vi "WorkorderHandler_LockedDataCache.vi"(0 "reference":T1, 2 "data in":T2, 5 "error in (no error)":errorcluster, 6 "action (read)":enum16{"push", "read", "pop"}(ring)=enum."read") -> (14 "reference dup":T1, 15 "found":bool, 16 "data out":T2, 19 "error out":errorcluster)   [LabVIEW 2011]
doc: "Stores locked data for read only access while the data is being modified."
uses:
  DataStructures/WorkorderHandler_ObjectReference.ctl
  DataStructures/WorkorderHandler_ObjectData.ctl
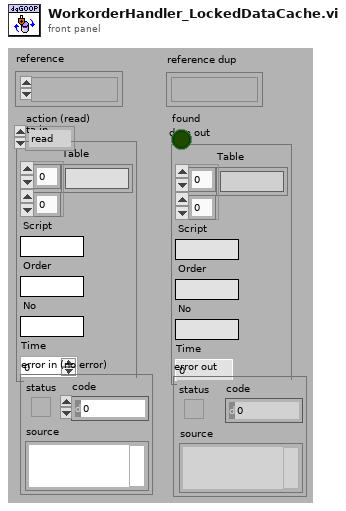
[diagram p1: front panel]
types:
  T1 = typedef "WorkorderHandler_ObjectReference.ctl" = refnum<k1>
  T2 = typedef "WorkorderHandler_ObjectData.ctl" = cluster{"Table":string[][], "Script":string, "Order":string, "No":string, "Time":dbl}
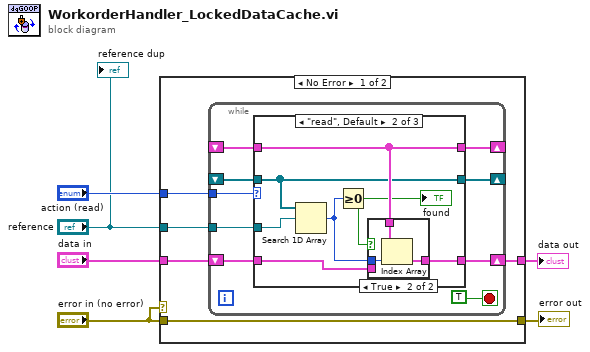
[diagram p0: block diagram]
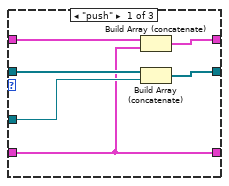
[diagram p2: hidden frame]
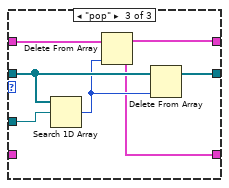
[diagram p4: hidden frame]
diagram:
  n1 = case shown="No Error" "error in (no error)" {
    tunnel: "action (read)" -> [w11 _]
    tunnel: "data in" -> [w10 w45]
    tunnel: "reference" -> [w8 _]
    tunnel: "error in (no error)" -> [w9 w46]
    tunnel: [w9 w46] -> w2
    tunnel: [w7 w45] -> w1
    frame No Error {
      n2 = while {
        shift-right: [w17] -> _
        shift-left: _ -> [w18]
        tunnel: w11 -> [w20]
        shift-right: [w15] -> _
        shift-left: _ -> [w16]
        tunnel: w8 -> [w14]
        shift-right: [w12] -> w7
        shift-left: w10 -> [w13]
        stop <- TRUE stop-if-true
        n3 = case shown="\"read\", Default" w20 {
          tunnel: w18 -> [w26 w32 w43]
          tunnel: [w25 w32 w42] -> w17
          tunnel: w16 -> [w24 w31 w41]
          tunnel: [w23 w31 w40] -> w15
          tunnel: w14 -> [w22 w33 w44]
          tunnel: w13 -> [w21 w27 _]
          tunnel: [w21 w29 w38] -> w12
          frame "push" {
            n4 = Build Array (concatenate)(w26, w21) -> (w25:T2[])
            n5 = Build Array (concatenate)(w24, w22) -> (w23:T1[])
          }
          frame "read", Default {
            n6 = Search 1D Array(1D array=w31, element=w33) -> (index of element=w30:i32)  [unwired: 1 out]
            n7 = Greater Or Equal To 0?(x=w30) -> (x >= 0?=w28:bool)
            "found" <- w28
            n8 = case shown="True" w28 {
              tunnel: w32 -> [_ w37]
              tunnel: w30 -> [_ w36]
              tunnel: [w34 w35] -> w29
              tunnel: w27 -> [w34 _]
              frame False {
              }
              frame True {
                n9 = Index Array(array=w37, index=w36) -> (element=w35:T2)
              }
            }
          }
          frame "pop" {
            n10 = Search 1D Array(1D array=w41, element=w44) -> (index of element=w39:i32)  [unwired: 1 out]
            n11 = Delete From Array(array=w43, index=w39) -> (deleted portion=w38:T2, array with subset deleted=w42:T2[])  [unwired: 1 in]
            n12 = Delete From Array(array=w41, index=w39) -> (array with subset deleted=w40:T1[])  [unwired: 1 in, 1 out]
          }
        }
      }
    }
    frame Error {
    }
  }
  "error out" <- w2
  "data out" <- w1
  "reference dup" <- "reference"
